vi "InitFile.vi"(8 "error in":errorcluster, 11 "INIFileClass in":refnum<class "INIFileClass.lvclass">) -> (0 "error out":errorcluster, 3 "INIFileClass out":refnum<class "INIFileClass.lvclass">)   [LabVIEW 2013, in "INIFileClass.lvclass"]
uses:
  INIFileClass.lvclass
  <vilib>/Utility/config.llb/NI_LVConfig.lvlib
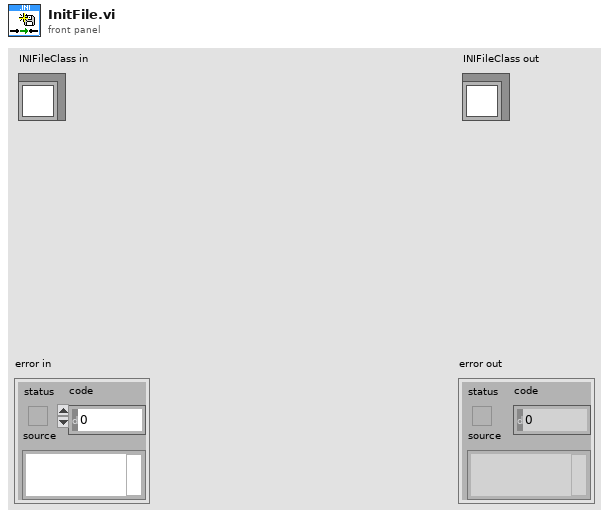
[diagram p1: front panel]
types:
  T1 = typedef "NI_LVConfig.lvlib/Config Data RefNum.ctl" = refnum<k1>
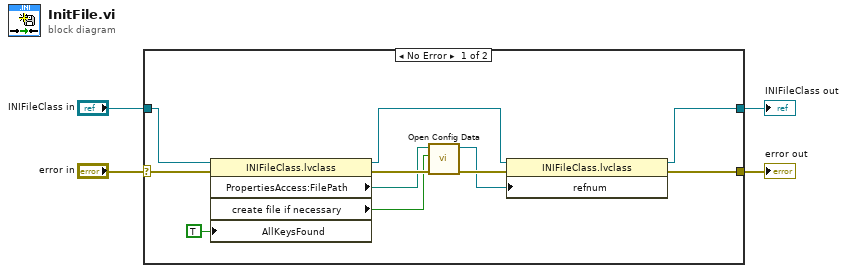
[diagram p0: block diagram]
diagram:
  n1 = case shown="No Error" "error in" {
    selector: "error in" -> [w14 w17]
    tunnel: [w7 w17] -> w3
    tunnel: [w5 w16] -> w1
    tunnel: "INIFileClass in" -> [w15 w16]
    frame No Error {
      n2 = property class="INIFileClass.lvclass"(reference=w15, error in=w14, "AllKeysFound"=TRUE) -> (reference out=w6:refnum<class "INIFileClass.lvclass">, error out=w13:errorcluster, "PropertiesAccess:FilePath"=w12:path, "create file if necessary"=w11:bool)
      n3 = call <vilib>:"Open Config Data.vi"("error in (no error)"=w13, "create file if necessary (T)"=w11, "configuration file path"=w12) -> ("error out"=w9:errorcluster, "refnum"=w8:T1)  [unwired: 6 in, 1 out]
      n4 = property class="INIFileClass.lvclass"(reference=w6, error in=w9, "refnum"=w8) -> (reference out=w5:refnum<class "INIFileClass.lvclass">, error out=w7:errorcluster)
    }
    frame Error {
    }
  }
  "error out" <- w3
  "INIFileClass out" <- w1
